vi "Unflatten Config.vi"(8 "error in (no error)":errorcluster, 11 "About Configuration File":path) -> (0 "error out":errorcluster, 2 "About Configuration":T1)   [LabVIEW 2013, in "About Screen Library.lvlib"]
uses:
  About Screen Library.lvlib
  Controls/Configuration Data.ctl
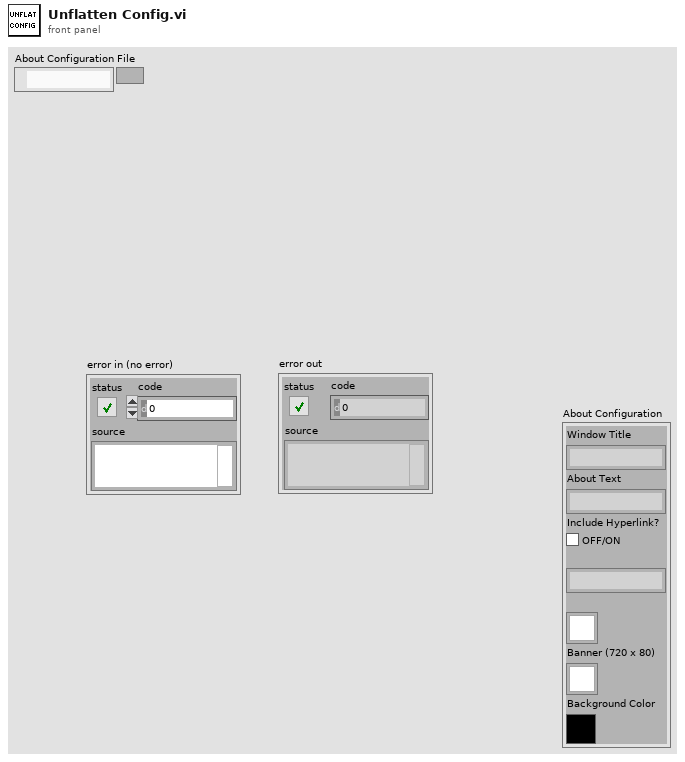
[diagram p1: front panel]
types:
  T1 = typedef "About Screen Library.lvlib/Configuration Data.ctl" = cluster{"Window Title":string, "About Text":string, "Include Hyperlink?":bool, "Hyperlink Path":string, "Logo (80 x 80)":picture, "Banner (720 x 80)":picture, "Background Color":u32}
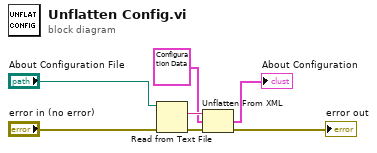
[diagram p0: block diagram]
diagram:
  n1 = Read from Text File(file (use dialog)="About Configuration File", error in="error in (no error)") -> (text=w6:string, error out=w1:errorcluster)  [unwired: 2 in, 2 out]
  n2 = Unflatten From XML(xml string=w6, type=T1 {"Window Title"="", "About Text"="", "Include Hyperlink?"=FALSE, "Hyperlink Path"="", "Logo (80 x 80)"=bytes[0], "Banner (720 x 80)"=bytes[0], "Background Color"=0} ("Configuration Data"), error in (no error)=w1) -> (value=→"About Configuration":T1, error out=→"error out":errorcluster)
